vi "基础24.vi"() -> ()   [LabVIEW 2014]
panel:
  in  "停止":bool
  out "波形图表":dynamicdata(graph)
  in  "布尔":bool
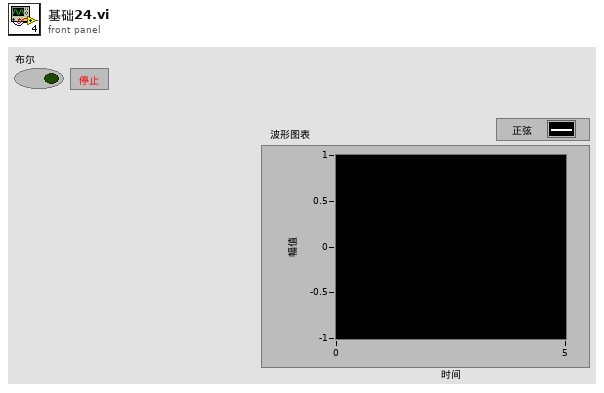
[diagram p1: front panel]
types:
  T1 = enum16{"open", "open or create", "create or replace", "create", "open (read-only)"}
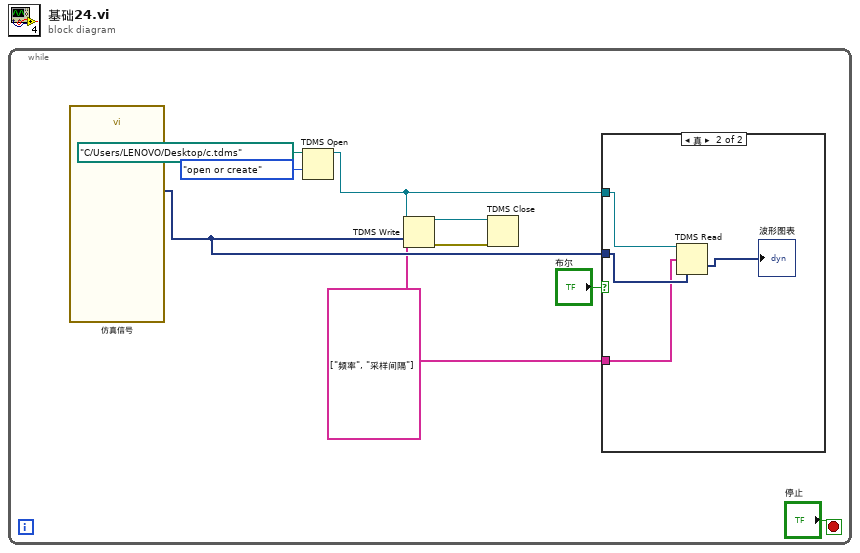
[diagram p0: block diagram]
diagram:
  n1 = while {
    stop <- "停止" stop-if-true
    w4 = string[] ["频率", "采样间隔"] ("通道名输入（无标题）")
    n2 = call "仿真信号"() -> ("正弦"=w6:dynamicdata)  [unwired: 14 in, 1 out]
    n3 = TDMS Open(10:T1."open or create" ("操作(0:open)"), 11:path "C:/Users/LENOVO/Desktop/c.tdms" ("文件路径")) -> (3:w5:refnum<k34>)  [unwired: 5 in, 1 out]
    n4 = TDMS Write(0:w5, 7:w4, 9:w6) -> (4:w2:refnum<k34>, 15:w1:errorcluster)  [unwired: 3 in, 2 out]
    n5 = TDMS Close(8:w1, 11:w2) -> ()  [unwired: 2 out]
    n6 = case shown="真" "布尔" {
      tunnel: w6 -> [_ w13]
      tunnel: w5 -> [_ w12]
      tunnel: w4 -> [_ w11]
      frame False {
      }
      frame True {
        n7 = TDMS Read(0:w12, 7:w11, 12:w13) -> (10:→"波形图表":dynamicdata)  [unwired: 5 in, 5 out]
      }
    }
  }
